vi "hw2.vi"(0 "Color Plane (Color Plane Extraction 1)":i32(ring) items=["Red", "Green", "Blue", "Hue", "Saturation", "Luminance", "Value", "Intensity"], 1 "Measurements (Measure 1)":i32[](array[numeric])=[3], 7 "error in":errorcluster) -> (27 "error out":errorcluster)   [LabVIEW 2014]
uses:
  <vilib>/Utility/file.llb/Write To Spreadsheet File (string).vi
  <vilib>/vision/NI_Vision_Development_Module.lvlib
panel:
  out "Image Out":T1(plugin-control)
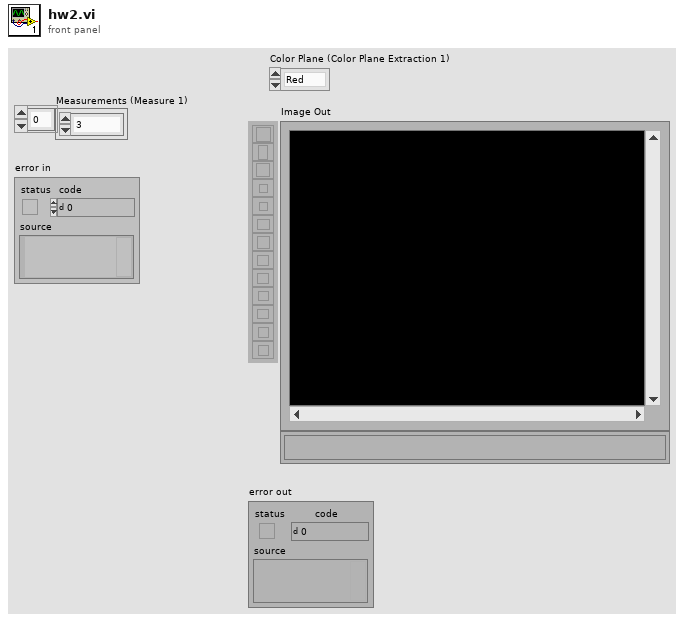
[diagram p1: front panel]
types:
  T1 = typedef "IMAQ Image.ctl" = refnum<image>
  T2 = cluster{"Global Rectangle":i32[], "Contours":cluster{"ID":enum32{"External", "Internal"}, "Type":u32, "Coordinates":i32[]}[]}[]
  T3 = typedef "Image Type" = u32
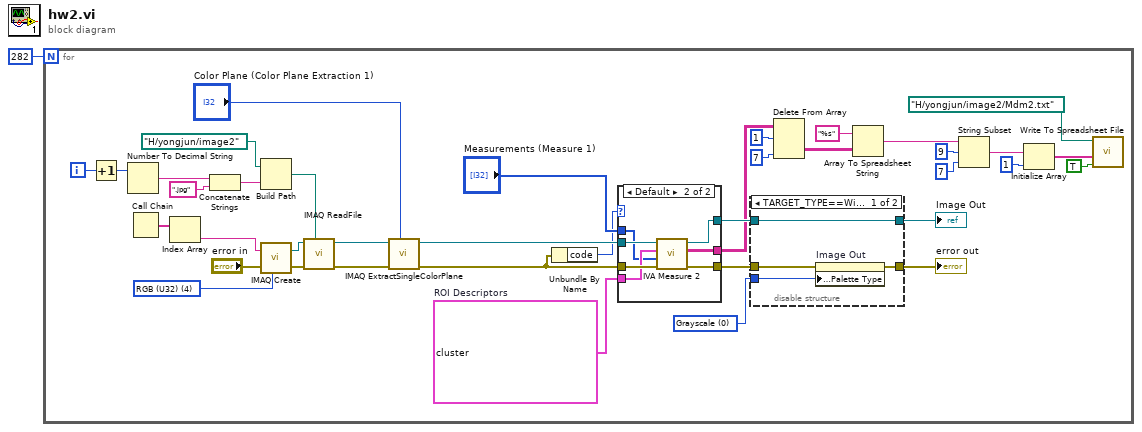
[diagram p0: block diagram]
diagram:
  n1 = for {
    N: 282 -> [_]
    i -> [w10]
    w22 = u32 0 items=["Grayscale", "Binary", "Gradient", "Rainbow", "Temperature", "User Defined"] ("Palette")
    w28 = T2 [{"Global Rectangle"=[23, 24, 181, 182], "Contours"=[{"ID"=enum."External", "Type"=3, "Coordinates"=[23, 24, 181, 182]}]}]  # ROI Descriptors
    w34 = T3 4 items=["Grayscale (U8)", "Grayscale (I16)", "Grayscale (SGL)", "Complex (CSG)", "RGB (U32)", "HSL (U32)", "RGB (U64)", "Grayscale (U16)"] ("Image Type")
    n2 = Increment(x=w10) -> (x+1=w9:i32)
    n3 = Number To Decimal String(number=w9) -> (decimal integer string=w17:string)  [unwired: 1 in]
    n4 = Call Chain() -> (call chain=w36:string[])
    n5 = Index Array(array=w36) -> (element=w35:string)  [unwired: 1 in]
    n6 = Concatenate Strings(w17, ".jpg") -> (w14:string)
    n7 = Build Path(base path=path "H:/yongjun/image2", name or relative path=w14) -> (appended path=w13:path)
    n8 = call "IMAQ Create"("Image Name"=w35, "Image Type"=w34, "error in (no error)"="error in") -> ("New Image"=w39:T1, "error out"=w38:errorcluster)  [unwired: 1 in, 1 out]
    n9 = call "IMAQ ReadFile"("File Path"=w13, "error in (no error)"=w38, "Image"=w39) -> ("error out"=w40:errorcluster, "Image Out"=w32:T1)  [unwired: 2 in, 5 out]
    n10 = call "IMAQ ExtractSingleColorPlane"("Color Plane"="Color Plane (Color Plane Extraction 1)", "error in (no error)"=w40, "Image Src"=w32) -> ("error out"=w31:errorcluster, "Image Dst Out"=w29:T1)  [unwired: 1 in, 6 out]
    n11 = Unbundle By Name(w31) -> ("code"=w26:i32)
    n12 = case shown="Default" w26 {
      tunnel: w31 -> [_ w54]
      tunnel: [_ w53] -> w30
      tunnel: w29 -> [w47 w52]
      tunnel: [w47 w51] -> w24
      tunnel: [_ w50] -> w20
      tunnel: w28 -> [_ w49]
      tunnel: "Measurements (Measure 1)" -> [_ w48]
      frame -1074396199, -1074396198 {
        # "Discard\nCoordinate\nSystem\nError"
      }
      frame Default {
        n13 = call <vilib>:"IVA Measure 2.vi"("error in (no error)"=w54, "Measurements"=w48, "ROI Descriptors"=w49, "Image In"=w52) -> ("error out"=w53:errorcluster, "Results"=w50:string[][], "Image Out"=w51:T1)  [unwired: 1 in, 4 out]
      }
    }
    n14 = disable-structure "Conditional Disable Structure" shown="TARGET_TYPE==Windows" {
      disable-tunnel: w30 -> [w44 w45]
      disable-tunnel: [w43 w45] -> w25
      disable-tunnel: w24 -> [w42 w46]
      disable-tunnel: [w42 w46] -> w23
      disable-tunnel: w22 -> [w41 _]
      frame condition #0 (active) {
        n15 = property on="Image Out" class="ImageControl"(error in=w44, "Palette:Palette Type"=w41) -> (error out=w43:errorcluster)  [unwired: 1 in, 1 out]
      }
      frame condition #1 {
      }
    }
    "error out" <- w25
    "Image Out" <- w23
    n16 = Delete From Array(array=w20, length=1, index (col)=7 ("disabled index (col)")) -> (deleted portion=w8:string[][])  [unwired: 1 in, 1 out]
    n17 = Array To Spreadsheet String(array=w8, 3:"%s") -> (spreadsheet string=w7:string)  [unwired: 1 in]
    n18 = String Subset(string=w7, offset (0)=9, length (rest)=7) -> (substring=w6:string)
    n19 = Initialize Array(w6, 1) -> (w5:string[])
    n20 = call-poly <vilib>:"Write To Spreadsheet File.vi"("append to file? (new file:F)"=TRUE, "1D data"=w5, "file path (dialog if empty)"=path "H:/yongjun/image2/Mdm2.txt") -> ()  [unwired: 5 in, 1 out]
  }
